vi "PicoScope2000SetupStreaming.vi"(0 "error in":errorcluster, 1 "Unit Info":T2, 2 "handle in":i16, 3 "Acquisition Settings":T1 {"Application Buffer Size" format="%#_6p"; "Time Units" items=["Nanoseconds (ns)", "Microseconds (us)", "Milliseconds (ms)", "Seconds (s)"]; "Overview Buffer Size" format="%#_6p"; "Max Samples" format="%#.6p"}, 4 "Buffer and Transfer Settings":T3 {"Down-Sample Mode" items=["None", "Aggregate", "Decimate", "Average"]; "Down Sample Ratio" step=1; "Samples" format="%#_6p"}, 5 "enabled array":i16[](array[numeric]), 10 "Pointers In":u64[][](array[numeric])) -> (11 "Pointer array":u64[][](array[numeric]), 14 "error out":errorcluster, 16 "handle out":i16, 17 "Sample Interval":u32, 19 "sampleIntervalTimeUnits":u32)   [LabVIEW 2009]
doc: "Set up the data buffers and calls RunStreaming to start the device streaming.\nData will be copied from the driver buffers into the corresponding application buffers using the wrapper dll."
uses:
  ps2000Wrap.dll
  ps2000.dll
panel:
  out "return":i16
  # "Overview Buffer Size is the size of the temporary buffers used to\nstore data before returning it to the application."
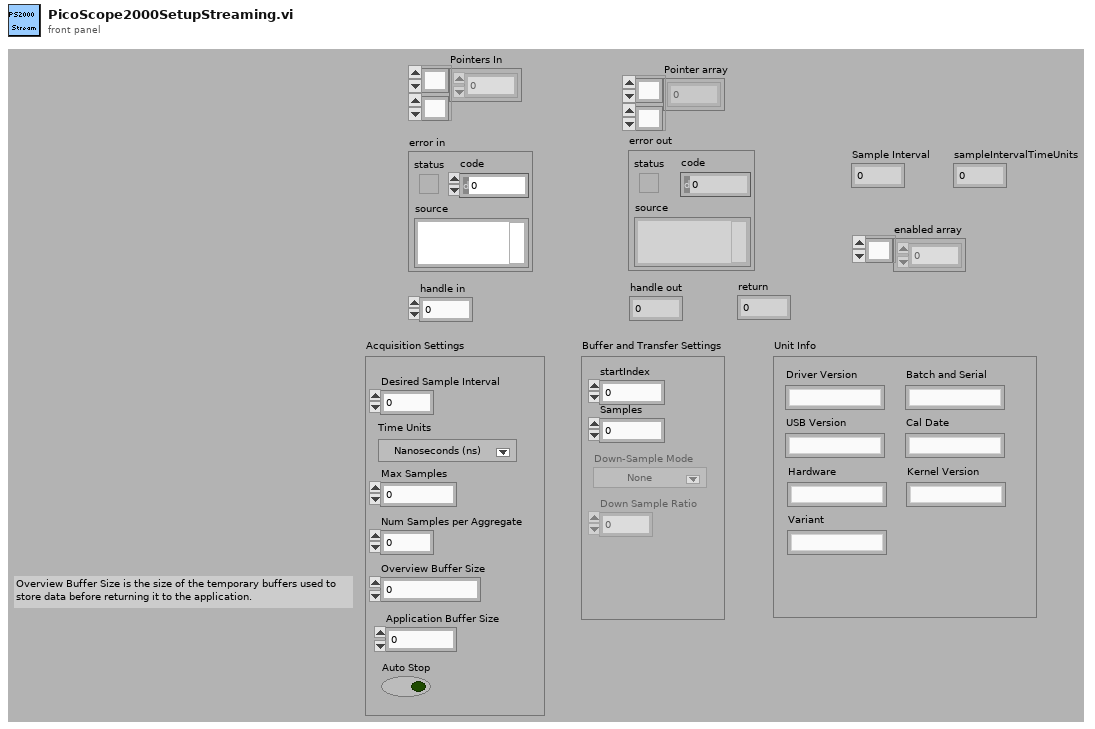
[diagram p1: front panel]
types:
  T1 = cluster{"Auto Stop":bool, "Desired Sample Interval":u32, "Max Samples":u32, "Num Samples per Aggregate":u32, "Overview Buffer Size":u32, "Time Units":u32, "Application Buffer Size":u32}
  T2 = cluster{"Driver Version":string, "USB Version":string, "Hardware":string, "Variant":string, "Batch and Serial":string, "Cal Date":string, "Kernel Version":string}
  T3 = cluster{"startIndex":u64, "Samples":u64, "Down Sample Ratio":u64, "Down-Sample Mode":u32}
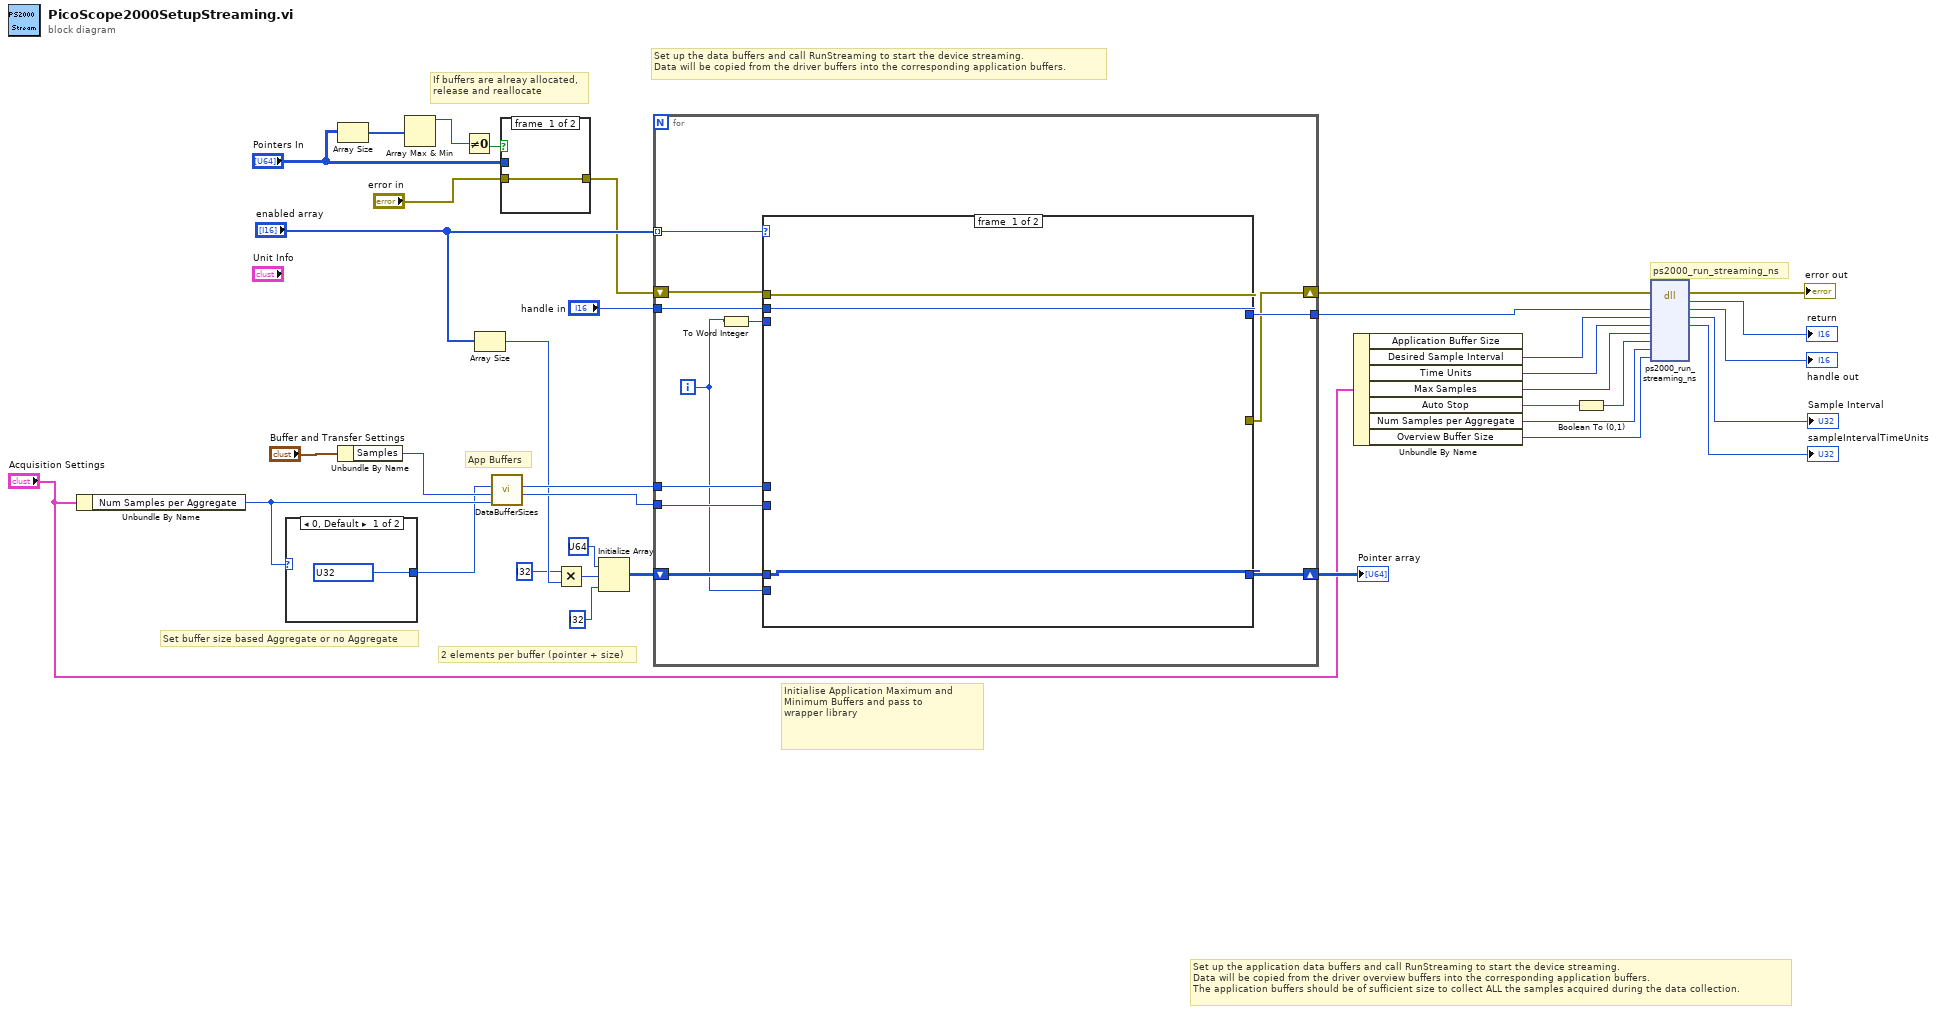
[diagram p0: block diagram]
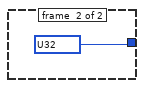
[diagram p2: hidden frame]
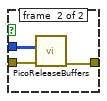
[diagram p3: hidden frame]
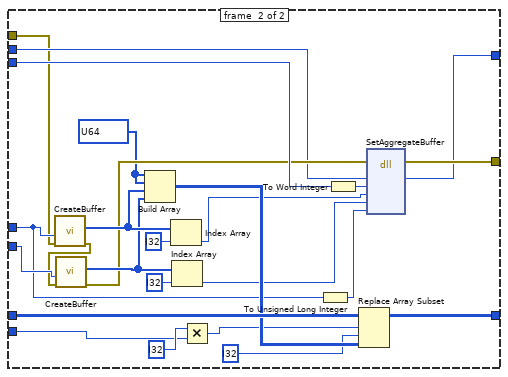
[diagram p4: hidden frame]
diagram:
  # "Set buffer size based Aggregate or no Aggregate"
  # "ps2000_run_streaming_ns"
  # "Set up the application data buffers and call RunStreaming to start the device streaming.\nData will be copied from the driver overview buffers into the corresponding application buffers.\nThe application buffers should be of sufficient size to collect ALL the samples acquired during the data collection."
  # "If buffers are alreay allocated,\nrelease and reallocate"
  # "2 elements per buffer (pointer + size)"
  # "App Buffers"
  # "Initialise Application Maximum and\nMinimum Buffers and pass to \nwrapper library"
  # "Set up the data buffers and call RunStreaming to start the device streaming.\nData will be copied from the driver buffers into the corresponding application buffers."
  n1 = Unbundle By Name("Acquisition Settings") -> ("Num Samples per Aggregate"=w2:u32)
  n2 = case shown="0, Default" w2 {
    tunnel: [w37 w38] -> w1
    frame #0 {
      w37 = u32 ? items=["RAW none", "None", "Aggregate", "Decimate", "Average"] ("Down-Sample Mode")
    }
    frame #1 {
      w38 = u32 ? items=["RAW none", "None", "Aggregate", "Decimate", "Average"] ("Down-Sample Mode")
    }
  }
  n3 = Array Size(array="Pointers In") -> (size(s)=w22:i32[])
  n4 = Unbundle By Name("Buffer and Transfer Settings") -> ("Samples"=w5:u64)
  n5 = Array Max & Min(array=w22) -> (max value=w21:i32)  [unwired: 3 out]
  n6 = Not Equal To 0?(x=w21) -> (x != 0?=w26:bool)
  n7 = Array Size(array="enabled array") -> (size(s)=w29:i32)
  n8 = call "DataBufferSizes.vi"("Down Sample Ratio"=w2, "Number of Samples"=w5, "Down-Sample Mode"=w1) -> ("min Buffer Size"=w35:i32, "Max Buffer Size"=w36:i32)  [unwired: 7 in]
  n9 = case shown="True" w26 {
    tunnel: "Pointers In" -> [_ w40]
    tunnel: "error in" -> [w39 w41]
    tunnel: [w39 w42] -> w7
    frame #0 {
    }
    frame #1 {
      n10 = call "PicoReleaseBuffers.vi"("error in (no error)"=w41, "Pointer array"=w40) -> ("error out"=w42:errorcluster)  [unwired: 8 in, 1 out]
    }
  }
  n11 = Multiply(x=i32 ?, y=w29) -> (x*y=w30:i32)
  n12 = Initialize Array(u64 ? ("element"), w30, i32 ? ("dimension size")) -> (w23:u64[][])
  n13 = for {
    tunnel: "enabled array" -> [w48] mode=indexing
    tunnel: "handle in" -> [w53]
    tunnel: w36 -> [w52]
    tunnel: w35 -> [w51]
    tunnel: [w49] -> w12
    shift-right: [w47] -> w13
    shift-left: w7 -> [w46]
    shift-right: [w50] -> w34
    shift-left: w23 -> [w45]
    i -> [w43]
    n14 = To Word Integer(number=w43) -> (16bit integer=w44:i16)
    n15 = case shown="1" w48 {
      tunnel: w53 -> [w55 w64]
      tunnel: w46 -> [w54 w57]
      tunnel: w44 -> [_ w68]
      tunnel: w52 -> [_ w67]
      tunnel: w51 -> [_ w79]
      tunnel: w45 -> [w56 w76]
      tunnel: [w56 w75] -> w50
      tunnel: w43 -> [_ w73]
      tunnel: [w55 w63] -> w49
      tunnel: [w54 w65] -> w47
      frame #0 {
      }
      frame #1 {
        w58 = u64[] ? ("Pointer and BufferSize")
        n16 = call "CreateBuffer.vi"("error in (no error)"=w57, "Buffer size"=w67) -> ("error out"=w69:errorcluster, "Pointer and BufferSize"=w78:u64[])  [unwired: 8 in]
        n17 = call "CreateBuffer.vi"("error in (no error)"=w69, "Buffer size"=w79) -> ("error out"=w66:errorcluster, "Pointer and BufferSize"=w77:u64[])  [unwired: 8 in]
        n18 = Build Array(w58, w58, w78, w77) -> (w72:u64[][])
        n19 = Index Array(array=w78, index=i32 ?) -> (element=w61:u64)
        n20 = Index Array(array=w77, index=i32 ?) -> (element=w59:u64)
        n21 = Multiply(x=i32 ?, y=w73) -> (x*y=w71:i32)
        n22 = To Unsigned Long Integer(number=w67) -> (unsigned 32bit integer=w60:u32)
        n23 = To Word Integer(number=w68) -> (16bit integer=w62:i16)
        n24 = Replace Array Subset(array=w76, new element=w72, index (row)=w71, index (col)=i32 ? ("disabled index (row)")) -> (w75:u64[][])
        n25 = dll-call lib="ps2000Wrap.dll" fn="SetAggregateBuffer"(error in=w66, "handle"=w64, "channel"=w62, "appMaxBuffer"=w61, "appMinBuffer"=w59, "bufferLength"=w60) -> (error out=w65:errorcluster, "handle"=w63:i16)  [unwired: 7 in, 1 out]
      }
    }
  }
  "Pointer array" <- w34
  n26 = Unbundle By Name("Acquisition Settings") -> ("Desired Sample Interval"=w18:u32, "Time Units"=w17:u32, "Max Samples"=w14:u32, "Auto Stop"=w19:bool, "Num Samples per Aggregate"=w6:u32, "Overview Buffer Size"=w15:u32)  [unwired: 1 out]
  n27 = Boolean To (0,1)(Boolean=w19) -> (0, 1=w16:i16)
  n28 = dll-call lib="PS2000.dll" fn="ps2000_run_streaming_ns"(error in=w13, "handle"=w12, "sample_interval"=w18, "time_units"=w17, "max_samples"=w14, "auto_stop"=w16, "noOfSamplesPerAggregate"=w6, "overview_buffer_size"=w15) -> (error out=→"error out":errorcluster, "return"=→"return":i16, "handle"=→"handle out":i16, "sample_interval"=→"Sample Interval":u32, "time_units"=→"sampleIntervalTimeUnits":u32)  [unwired: 6 in, 1 out]
